vi "check info.vi"   [LabVIEW 2018]
uses:
  Vision info.vi
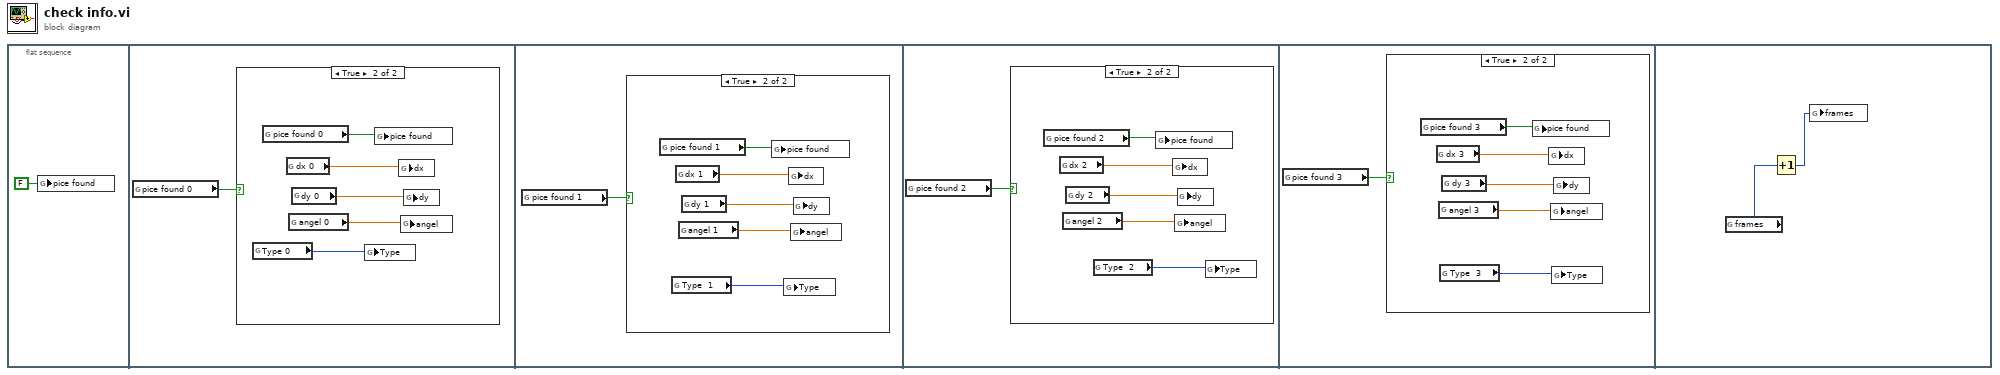
[diagram p0: block diagram]
diagram:
  n1 = flat-sequence {
    frame #0 {
      n2 = global write "Vision info.vi" "pice found"(FALSE ("pice found")) -> ()
    }
    frame #1 {
      n3 = global read "Vision info.vi" "pice found 0"() -> (w2:bool)
      n4 = case shown="True" w2 {
        frame False {
        }
        frame True {
          n5 = global read "Vision info.vi" "Type 0"() -> (w3:enum16{"Z", "I", "O", "S", "L", "J", "T", "N"})
          n6 = global read "Vision info.vi" "pice found 0"() -> (w7:bool)
          n7 = global read "Vision info.vi" "dx 0"() -> (w6:dbl)
          n8 = global read "Vision info.vi" "angel 0"() -> (w4:dbl)
          n9 = global read "Vision info.vi" "dy 0"() -> (w5:dbl)
          n10 = global write "Vision info.vi" "Type"(w3) -> ()
          n11 = global write "Vision info.vi" "pice found"(w7) -> ()
          n12 = global write "Vision info.vi" "dx"(w6) -> ()
          n13 = global write "Vision info.vi" "angel"(w4) -> ()
          n14 = global write "Vision info.vi" "dy"(w5) -> ()
        }
      }
    }
    frame #2 {
      n15 = global read "Vision info.vi" "pice found 1"() -> (w8:bool)
      n16 = case shown="True" w8 {
        frame False {
        }
        frame True {
          n17 = global read "Vision info.vi" "pice found 1"() -> (w13:bool)
          n18 = global read "Vision info.vi" "Type  1"() -> (w9:enum16{"Z", "I", "O", "S", "L", "J", "T", "N"})
          n19 = global read "Vision info.vi" "dx 1"() -> (w12:dbl)
          n20 = global read "Vision info.vi" "angel 1"() -> (w10:dbl)
          n21 = global read "Vision info.vi" "dy 1"() -> (w11:dbl)
          n22 = global write "Vision info.vi" "pice found"(w13) -> ()
          n23 = global write "Vision info.vi" "Type"(w9) -> ()
          n24 = global write "Vision info.vi" "dx"(w12) -> ()
          n25 = global write "Vision info.vi" "angel"(w10) -> ()
          n26 = global write "Vision info.vi" "dy"(w11) -> ()
        }
      }
    }
    frame #3 {
      n27 = global read "Vision info.vi" "pice found 2"() -> (w14:bool)
      n28 = case shown="True" w14 {
        frame False {
        }
        frame True {
          n29 = global read "Vision info.vi" "pice found 2"() -> (w19:bool)
          n30 = global read "Vision info.vi" "dx 2"() -> (w18:dbl)
          n31 = global read "Vision info.vi" "angel 2"() -> (w16:dbl)
          n32 = global read "Vision info.vi" "dy 2"() -> (w17:dbl)
          n33 = global read "Vision info.vi" "Type  2"() -> (w15:enum16{"Z", "I", "O", "S", "L", "J", "T", "N"})
          n34 = global write "Vision info.vi" "pice found"(w19) -> ()
          n35 = global write "Vision info.vi" "dx"(w18) -> ()
          n36 = global write "Vision info.vi" "angel"(w16) -> ()
          n37 = global write "Vision info.vi" "dy"(w17) -> ()
          n38 = global write "Vision info.vi" "Type"(w15) -> ()
        }
      }
    }
    frame #4 {
      n39 = global read "Vision info.vi" "pice found 3"() -> (w20:bool)
      n40 = case shown="True" w20 {
        frame False {
        }
        frame True {
          n41 = global read "Vision info.vi" "pice found 3"() -> (w25:bool)
          n42 = global read "Vision info.vi" "dx 3"() -> (w24:dbl)
          n43 = global read "Vision info.vi" "angel 3"() -> (w22:dbl)
          n44 = global read "Vision info.vi" "Type  3"() -> (w21:enum16{"Z", "I", "O", "S", "L", "J", "T", "N"})
          n45 = global read "Vision info.vi" "dy 3"() -> (w23:dbl)
          n46 = global write "Vision info.vi" "pice found"(w25) -> ()
          n47 = global write "Vision info.vi" "dx"(w24) -> ()
          n48 = global write "Vision info.vi" "angel"(w22) -> ()
          n49 = global write "Vision info.vi" "Type"(w21) -> ()
          n50 = global write "Vision info.vi" "dy"(w23) -> ()
        }
      }
    }
    frame #5 {
      n51 = global read "Vision info.vi" "frames"() -> (w27:i32)
      n52 = Increment(x=w27) -> (x+1=w26:i32)
      n53 = global write "Vision info.vi" "frames"(w26) -> ()
    }
  }
